vi "Main_API.vi"() -> ()   [LabVIEW 2018]
uses:
  <vilib>/httpClient/LabVIEWHTTPClient.lvlib
panel:
  in  "Blank Button":bool
  in  "stop":bool
  out "Temperature":string
  in  "CITY Box":string(combo)="Taipei"
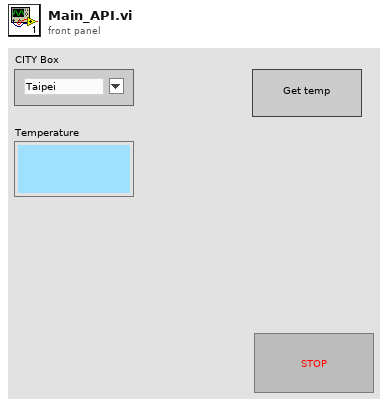
[diagram p1: front panel]
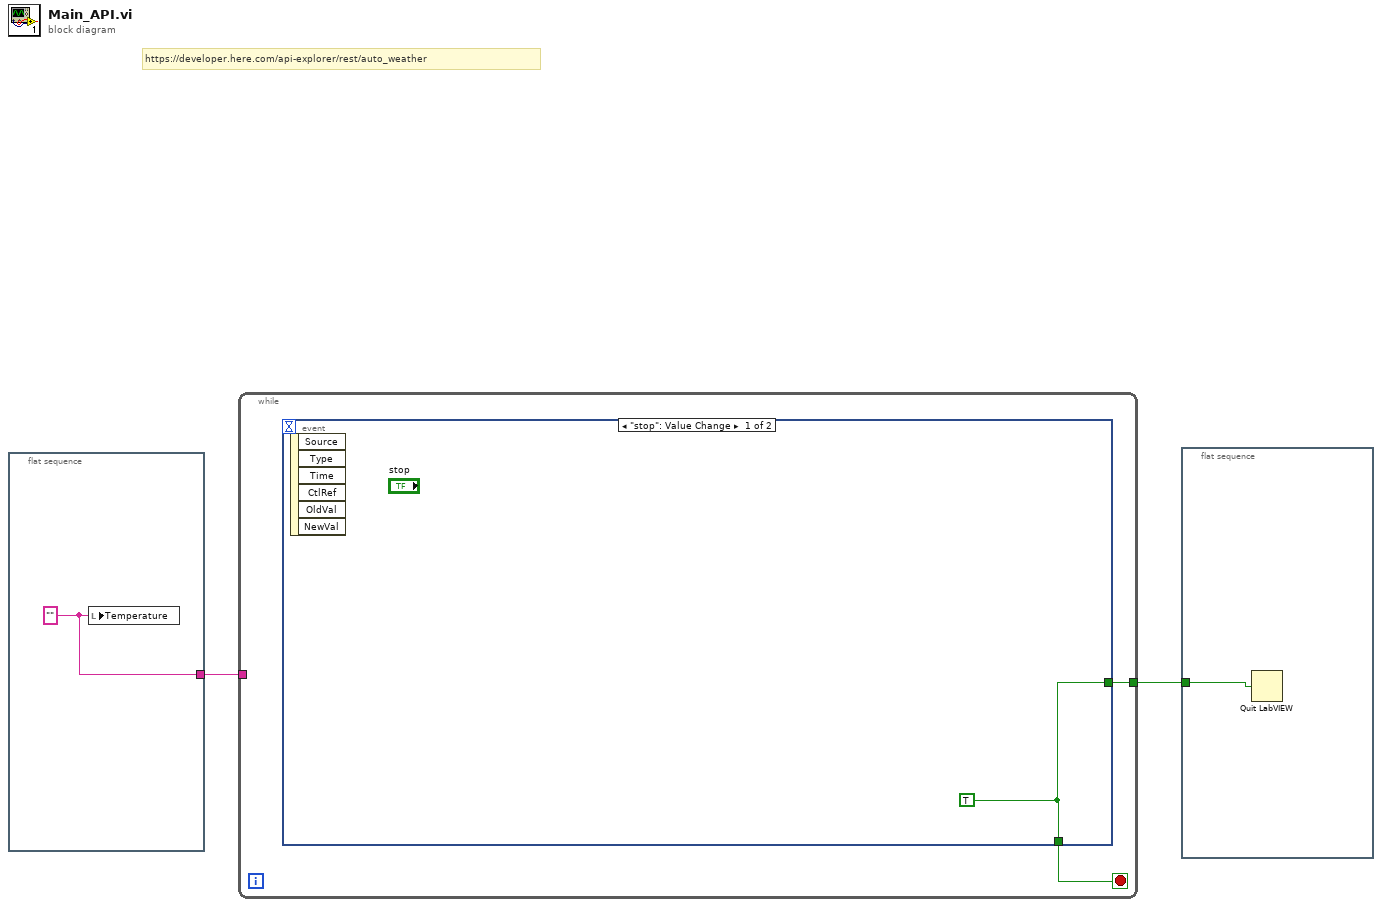
[diagram p0: block diagram]
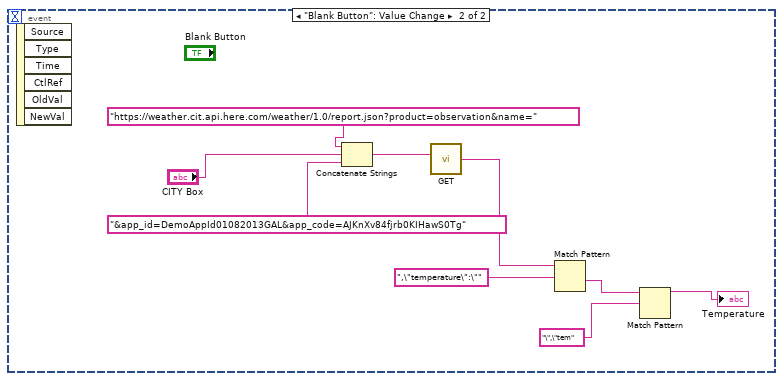
[diagram p2: hidden frame]
diagram:
  # "https://developer.here.com/api-explorer/rest/auto_weather"
  n1 = flat-sequence {
    tunnel: [w3] -> w2
    frame #0 {
      w3 = "" ("Temperature")
      n2 = local write "Temperature"(w3) -> ()
    }
  }
  n3 = while {
    tunnel: w2 -> [_]
    tunnel: [w4] -> w1
    stop <- w5 stop-if-true
    n4 = event shown="[0] \"stop\": Value Change" {
      selector: _ -> [_ _]
      dyn-events: _ -> [_ _]
      timeout: _ -> [_ _]
      tunnel: [w6 _] -> w5
      tunnel: [w6 _] -> w4
      event "stop": Value Change {
        w6 = TRUE
        n5 = event-data() -> ()  [unwired: 1 in, 6 out]
      }
      event "Blank Button": Value Change {
        n6 = event-data() -> ()  [unwired: 1 in, 6 out]
        n7 = Concatenate Strings("https://weather.cit.api.here.com/weather/1.0/report.json?product=observation&name=", "CITY Box", "&app_id=DemoAppId01082013GAL&app_code=AJKnXv84fjrb0KIHawS0Tg" ("string")) -> (w12:string)
        n8 = call <vilib>:"GET.vi"("url"=w12) -> ("body"=w13:string)  [unwired: 11 in, 3 out]
        n9 = Match Pattern(string=w13, regular expression=",\"temperature\":\"") -> (after substring=w14:string)  [unwired: 1 in, 3 out]
        n10 = Match Pattern(string=w14, regular expression="\",\"tem") -> (before substring=→"Temperature":string)  [unwired: 1 in, 3 out]
      }
    }
  }
  n11 = flat-sequence {
    tunnel: w1 -> [w16]
    frame #0 {
      n12 = Quit LabVIEW(quit? (T)=w16) -> ()
    }
  }
